vi "FlushMessages.vi"(8 "error in (no error)":errorcluster, 11 "zmq_socket in":refnum<class "zmq_socket.lvclass">) -> (0 "error out":errorcluster, 3 "zmq_socket out":refnum<class "zmq_socket.lvclass">)   [LabVIEW 2017]
uses:
  <vilib>/addons/zeromq/zmq_socket.lvclass
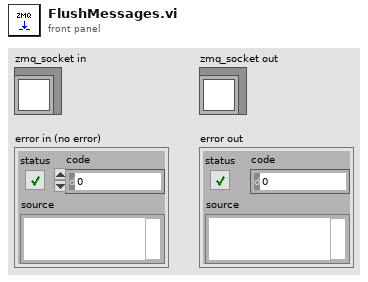
[diagram p1: front panel]
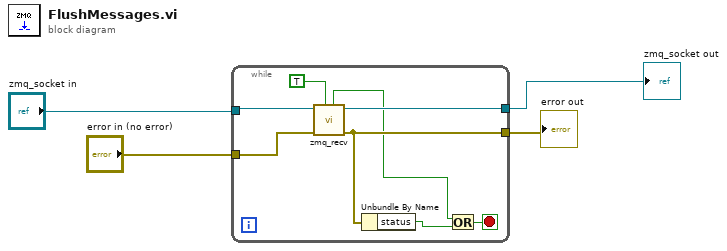
[diagram p0: block diagram]
diagram:
  n1 = while {
    tunnel: "zmq_socket in" -> [w11]
    tunnel: "error in (no error)" -> [w10]
    tunnel: [w8] -> w4
    tunnel: [w9] -> w3
    stop <- w7 stop-if-true
    n2 = call <vilib>:"zmq_recv.vi"("no block? (F)"=TRUE, "error in"=w10, "socket in"=w11) -> ("error out"=w8:errorcluster, "socket out"=w9:refnum<class "zmq_socket.lvclass">, "timeout?"=w6:bool)  [unwired: 2 in, 2 out]
    n3 = Unbundle By Name(w8) -> ("status"=w5:bool)
    n4 = Or(x=w6, y=w5) -> (x .or. y?=w7:bool)
  }
  "error out" <- w4
  "zmq_socket out" <- w3
